vi "Análise de temperatura.vi"() -> ()   [LabVIEW 2018]
uses:
  <vilib>/Analysis/NI_AALBase.lvlib
  <vilib>/Analysis/NI_AALPro.lvlib
panel:
  out "Polynomial Coefficients":dbl[](array[numeric]) format="%#_2f"
  out "Waveform Graph":dbl[][](graph)
  in  "polynomial order":i32=2 format="%.2f"
  out "variance":dbl format="%.2f"
  out "standard deviation":dbl format="%.2f"
  out "mean":dbl format="%.2f"
  out "min value":dbl format="%#_2f"
  out "max value":dbl format="%#_2f"
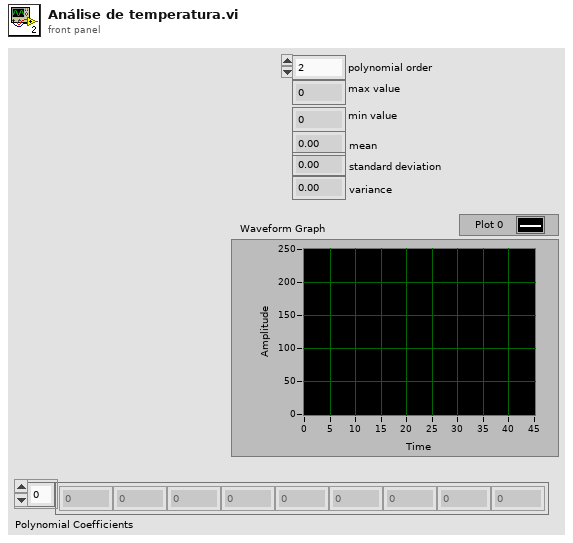
[diagram p1: front panel]
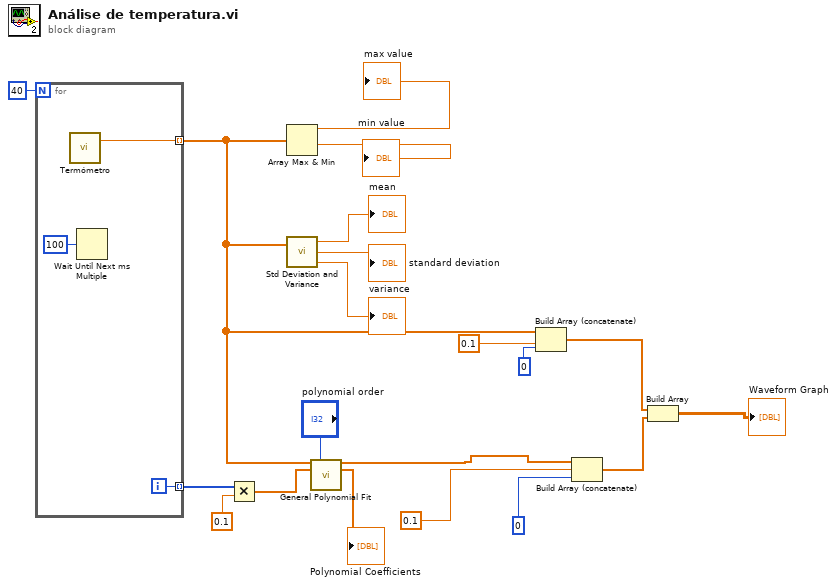
[diagram p0: block diagram]
diagram:
  n1 = for {
    N: 40 -> [_]
    tunnel: [w23] -> w10 mode=indexing
    tunnel: [w21] -> w14 mode=indexing
    i -> [w21]
    n2 = call "Termómetro.vi"() -> ("Thermometer"=w23:dbl)  [unwired: 3 in]
    n3 = Wait Until Next ms Multiple(millisecond multiple=u32 100) -> ()  [unwired: 1 out]
  }
  n4 = Multiply(x=w14, y=0.1) -> (x*y=w12:dbl[])
  n5 = Array Max & Min(array=w10) -> (max value=→"max value":dbl, min value=→"min value":dbl)  [unwired: 2 out]
  n6 = call <vilib>:"Std Deviation and Variance.vi"("X"=w10) -> ("mean"=→"mean":dbl, "standard deviation"=→"standard deviation":dbl, "variance"=→"variance":dbl)  [unwired: 1 in]
  n7 = call <vilib>:"General Polynomial Fit.vi"("Y"=w10, "polynomial order"="polynomial order", "X"=w12) -> ("Best Polynomial Fit"=w6:dbl[], "Polynomial Coefficients"=→"Polynomial Coefficients":dbl[])  [unwired: 9 in, 2 out]
  n8 = Build Array (concatenate)(w10, 0.1, 0) -> (w7:dbl[])
  n9 = Build Array (concatenate)(w6, 0.1, 0) -> (w3:dbl[])
  n10 = Build Array(w7, w3) -> (→"Waveform Graph":dbl[][])
